vi "TermoparRef2.vi"() -> ()   [LabVIEW 2014]
panel:
  in  "InputData":dbl
  in  "Offset2":dbl step=0.01 format="%#_2f"
  in  "Offset1":dbl step=0.1 format="%#_3f"
  out "LM35 temperature (degC)":dbl format="%#_3f"
  out "Emf(Cold - mV)":dbl
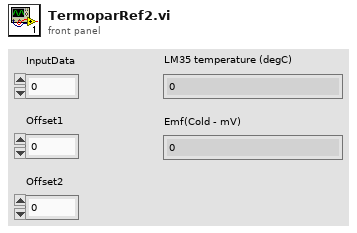
[diagram p1: front panel]
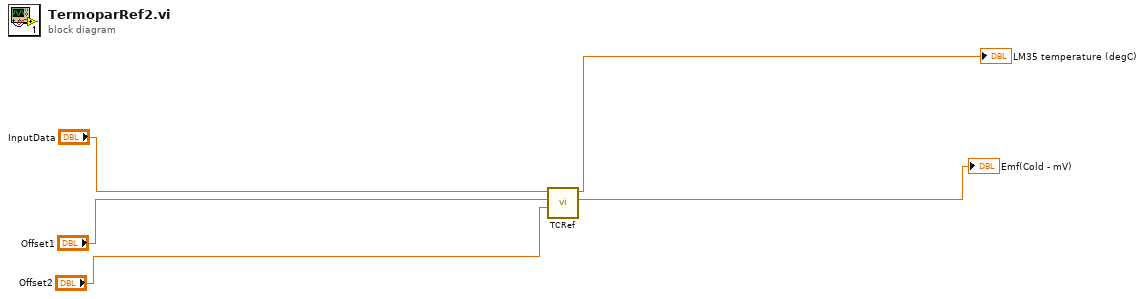
[diagram p0: block diagram]
diagram:
  n1 = call "TCRef.vi"("Offset2"="Offset2", "Offset1"="Offset1", "InputData"="InputData") -> ("Numeric"=→"Emf(Cold - mV)":dbl, "Numeric 2"=→"LM35 temperature (degC)":dbl)  [unwired: 7 in]
